vi "populate_users.vi"(7 "set combobox grayed out? (F)":bool, 8 "error in (no error)":errorcluster, 10 "user name":string, 11 "ref username in":refnum<vi>) -> (0 "error out":errorcluster, 2 "user names":string[](array[string]))   [LabVIEW 2010, in "XUserDropdown.xctl"]
doc: "If reference is wired, the default username is taken. This is useful for a test.vi."
uses:
  XUserDropdown.xctl
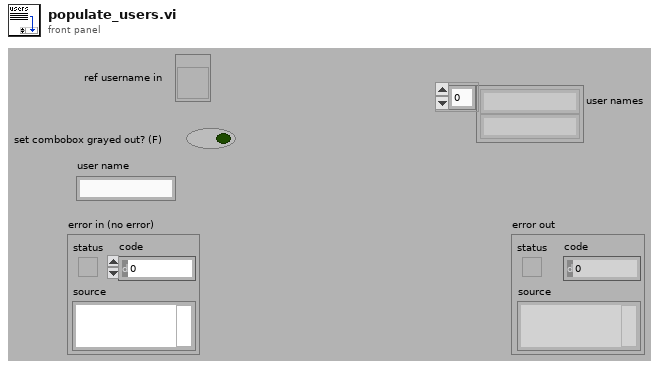
[diagram p1: front panel]
types:
  T1 = enum8{"Enabled", "Disabled", "Disabled and Grayed Out"}
  T2 = typedef "configuration_paths_cluster.ctl" = cluster{"base folder":path, "base folder for user":path, "component folder":path, "component file path":path, "main folder":path, "main file":path}
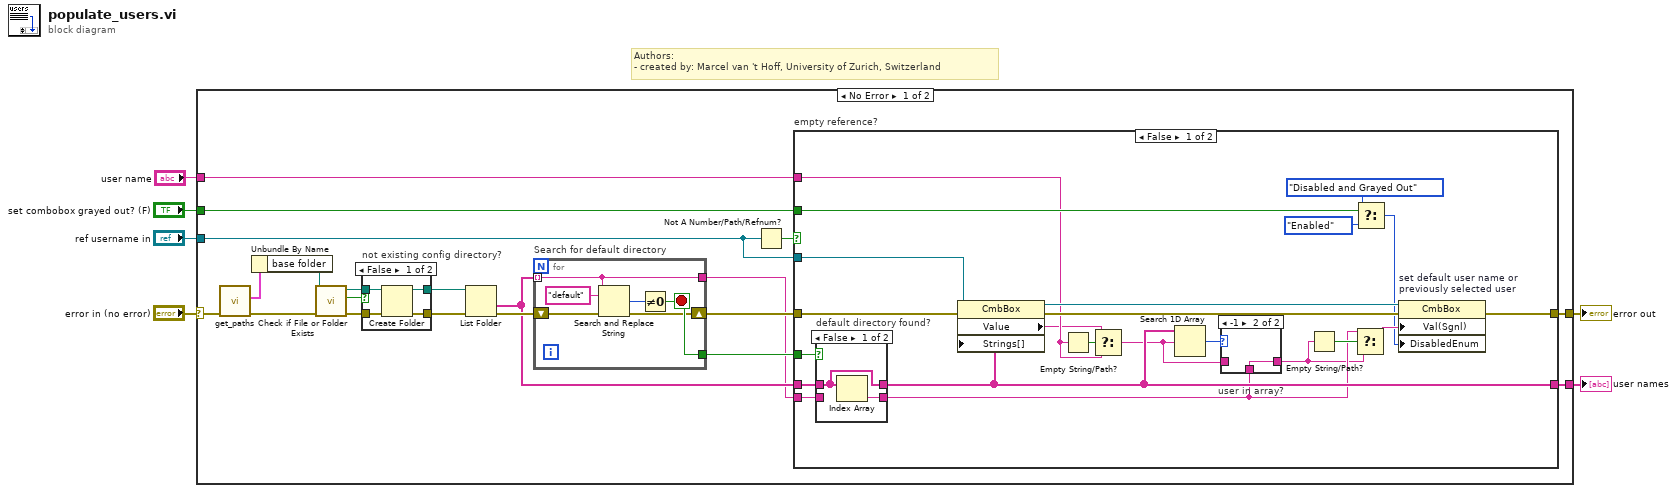
[diagram p0: block diagram]
diagram:
  # "Authors: \n- created by: Marcel van 't Hoff, University of Zurich, Switzerland"
  n1 = case shown="No Error" "error in (no error)" {
    selector: "error in (no error)" -> [w16 w69]
    tunnel: [w24 w69] -> w5
    tunnel: [w19 _] -> w4
    tunnel: "ref username in" -> [w25 _]
    tunnel: "set combobox grayed out? (F)" -> [w18 _]
    tunnel: "user name" -> [w14 _]
    frame No Error {
      n2 = call "get_paths.vi"("error in (no error)"=w16) -> ("error out"=w12:errorcluster, "configuration paths"=w17:T2)  [unwired: 7 in, 2 out]
      n3 = Unbundle By Name(w17) -> ("base folder"=w13:path)
      n4 = call <vilib>:"Check if File or Folder Exists.vi"("error in (no error)"=w12, "path"=w13) -> ("error out"=w9:errorcluster, "file or folder exists?"=w11:bool, "dup path"=w10:path)  [unwired: 7 in]
      n5 = case "not existing config directory?" shown="False" w11 {
        tunnel: w10 -> [w30 w31]
        tunnel: w9 -> [w29 w32]
        tunnel: [w28 w32] -> w8
        tunnel: [w27 w31] -> w7
        frame False {
          n6 = Create Folder(path (use dialog)=w30, error in=w29) -> (created path=w27:path, error out=w28:errorcluster)  [unwired: 1 in, 1 out]
        }
        frame True {
        }
      }
      n7 = List Folder(path=w7, error in=w8) -> (folder names=w20:string[], error out=w23:errorcluster)  [unwired: 2 in, 2 out]
      n8 = for "Search for default directory" {
        tunnel: w20 -> [w33] mode=indexing
        tunnel: [w35] -> w21
        shift-right: [w34] -> w22
        shift-left: w23 -> [w36]
        tunnel: [w33] -> w15
        stop <- w35 stop-if-true
        n9 = Search and Replace String(input string=w33, search string="default", error in=w36) -> (number of replacements=w37:i32, error out=w34:errorcluster)  [unwired: 5 in, 2 out]
        n10 = Not Equal To 0?(x=w37) -> (x != 0?=w35:bool)
      }
      n11 = Not A Number/Path/Refnum?(number/path/refnum=w25) -> (NaN/Path/Refnum?=w26:bool)
      n12 = case "empty reference?" shown="False" w26 {
        tunnel: w25 -> [w55 _]
        tunnel: w22 -> [w57 w68]
        tunnel: [w54 w68] -> w24
        tunnel: w21 -> [w60 _]
        tunnel: w20 -> [w59 w67]
        tunnel: [w43 w67] -> w19
        tunnel: w18 -> [w50 _]
        tunnel: w15 -> [w53 _]
        tunnel: w14 -> [w45 _]
        frame False {
          n13 = case "default directory found?" shown="False" w60 {
            tunnel: [w64 w65] -> w41
            tunnel: w59 -> [w63 w66]
            tunnel: [w63 w66] -> w43
            tunnel: w53 -> [_ w65]
            frame False {
              n14 = Index Array(array=w63) -> (element=w64:string)  [unwired: 1 in]
            }
            frame True {
            }
          }
          n15 = property class="CmbBox"(reference=w55, error in=w57, "Strings[]"=w43) -> (reference out=w58:refnum<vi>, error out=w56:errorcluster, "Value"=w44:string)
          n16 = Empty String/Path?(string/path=w45) -> (empty?=w46:bool)
          n17 = Select(t=w44, s=w46, f=w45) -> (s? t:f=w40:string)
          n18 = Search 1D Array(1D array=w43, element=w40) -> (index of element=w42:i32)  [unwired: 1 in]
          n19 = case "user in array?" shown="-1" w42 {
            tunnel: w40 -> [w61 _]
            tunnel: [w61 w62] -> w39
            tunnel: w41 -> [_ w62]
            frame Default {
            }
            frame -1 {
            }
          }
          n20 = Empty String/Path?(string/path=w39) -> (empty?=w52:bool)
          n21 = Select(t=w41, s=w52, f=w39) -> (s? t:f=w51:string)
          n22 = Select(t=T1."Disabled and Grayed Out" ("Disabled"), s=w50, f=T1."Enabled" ("Disabled")) -> (s? t:f=w49:T1)
          n23 = property on="set default user name or previously selected user" class="CmbBox"(reference=w58, error in=w56, "Val(Sgnl)"=w51, "DisabledEnum"=w49) -> (error out=w54:errorcluster)  [unwired: 1 out]
        }
        frame True {
        }
      }
    }
    frame Error {
    }
  }
  "error out" <- w5
  "user names" <- w4
